vi "Read Last Image.vi"(8 "error in (no error)":errorcluster, 11 "CCDCamera in":refnum<class "CCDCamera.lvclass">) -> (0 "error out":errorcluster, 1 "Last Image":string, 2 "Last Image Path":string, 3 "CCDCamera out":refnum<class "CCDCamera.lvclass">)   [LabVIEW 2018, in "CCDCamera.lvclass"]
doc: "This VI reads the name of the last image acquired."
uses:
  CCDCamera.lvclass
  CCDCamera.lvclass/CCDCamera.ctl
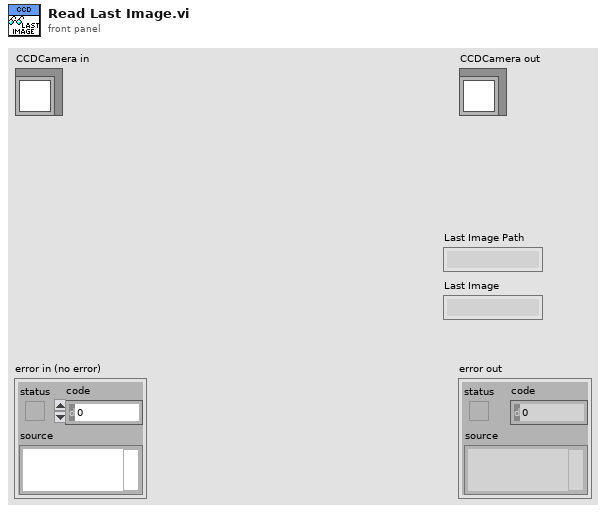
[diagram p1: front panel]
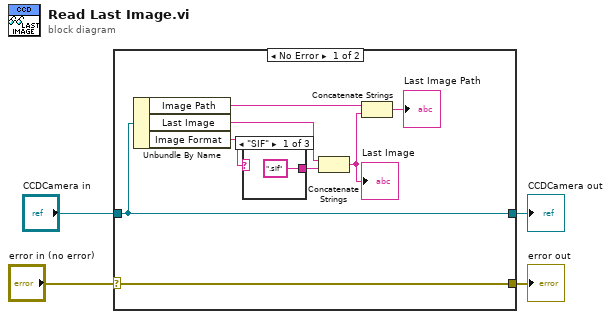
[diagram p0: block diagram]
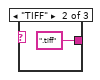
[diagram p2: hidden frame]
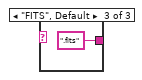
[diagram p3: hidden frame]
diagram:
  n1 = case shown="No Error" "error in (no error)" {
    selector: "error in (no error)" -> [w12 w17]
    tunnel: [w12 w17] -> w3
    tunnel: [w11 w16] -> w1
    tunnel: "CCDCamera in" -> [w11 w16]
    frame No Error {
      n2 = Unbundle By Name(w11) -> ("Image Path"=w5:string, "Last Image"=w9:string, "Image Format"=w10:string)
      n3 = case shown="\"SIF\"" w10 {
        tunnel: [".sif" ("string") ".tiff" ("string") ".fits" ("string")] -> w8
        frame "SIF" {
        }
        frame "TIFF" {
        }
        frame "FITS", Default {
        }
      }
      n4 = Concatenate Strings(w9, w8) -> (w6:string)
      "Last Image" <- w6
      n5 = Concatenate Strings(w5, w6) -> (→"Last Image Path":string)
    }
    frame Error {
    }
  }
  "error out" <- w3
  "CCDCamera out" <- w1
